vi "InitGraphsTableDisplay.vi"(11 "DisplayGraphsTable_In":refnum<vi>) -> (3 "DisplayGraphsTable_Out":refnum<vi>)   [LabVIEW 2013]
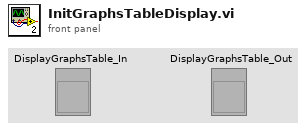
[diagram p1: front panel]
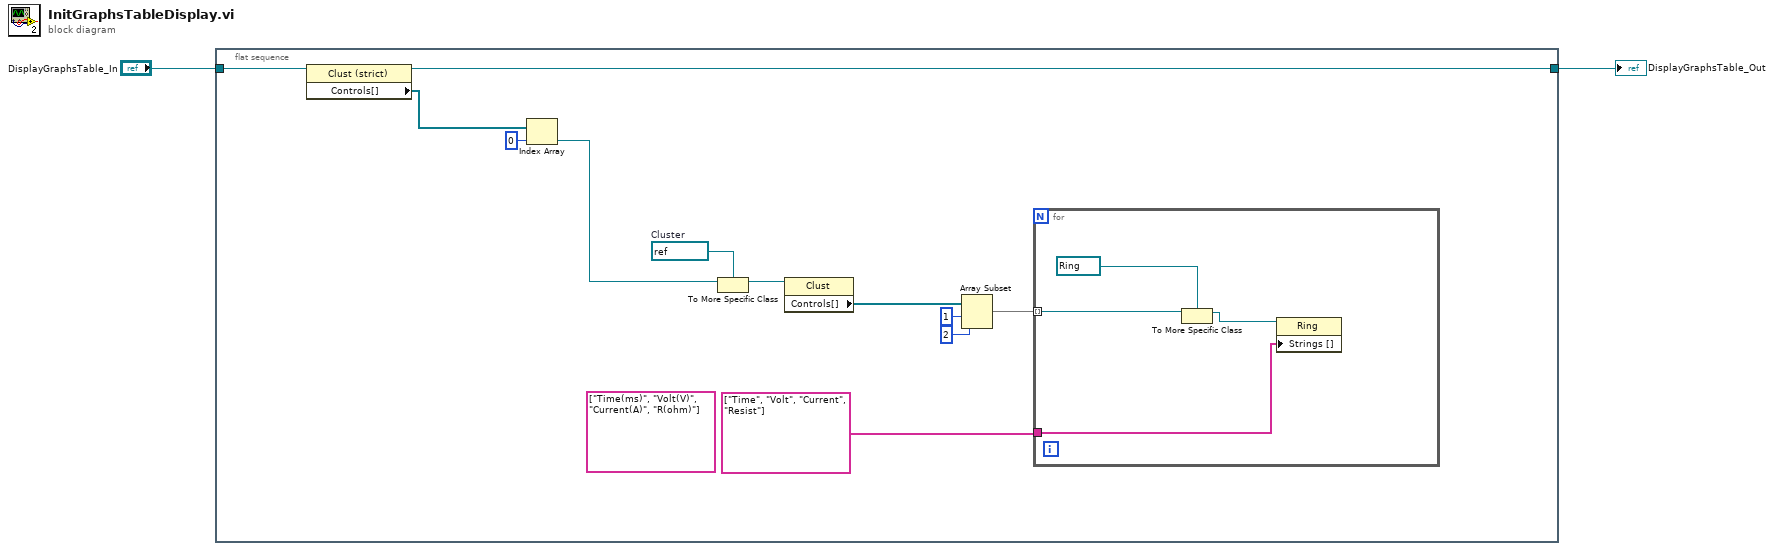
[diagram p0: block diagram]
diagram:
  n1 = flat-sequence {
    tunnel: [w5] -> w2
    tunnel: "DisplayGraphsTable_In" -> [w6]
    frame #0 {
      w4 = refnum<vi> refnum  # Cluster
      (unwired) string[] ["Time(ms)", "Volt(V)", "Current(A)", "R(ohm)"]
      n2 = property class="Clust (strict)"(reference=w6) -> (reference out=w5:refnum<vi>, "Controls[]"=w14:refnum<vi>[])  [unwired: 1 in, 1 out]
      n3 = Index Array(array=w14, index=0) -> (element=w12:refnum<vi>)
      n4 = To More Specific Class(target class=w4, reference=w12) -> (specific class reference=w11:refnum<vi>)  [unwired: 1 in, 1 out]
      n5 = property class="Clust"(reference=w11) -> ("Controls[]"=w10:refnum<vi>[])  [unwired: 1 in, 2 out]
      n6 = Array Subset(array=w10, index=1, length=2) -> (w7:refnum<vi>[])
      n7 = for {
        tunnel: w7 -> [w18] mode=indexing
        tunnel: string[] ["Time", "Volt", "Current", "Resist"] -> [w15]
        n8 = To More Specific Class(target class=refnum<vi> refnum ("X is"), reference=w18) -> (specific class reference=w16:refnum<vi>)  [unwired: 1 in, 1 out]
        n9 = property class="Ring"(reference=w16, "Strings []"=w15) -> ()  [unwired: 1 in, 2 out]
      }
    }
  }
  "DisplayGraphsTable_Out" <- w2
